vi "prepAO_tt.vi"() -> ()   [LabVIEW 2015]
uses:
  <vilib>/DAQmx/write.llb/DAQmx Write (Analog 1D Wfm NChan NSamp).vi
  <vilib>/DAQmx/create/channels.llb/DAQmx Create Channel (AO-Voltage-Basic).vi
  <vilib>/DAQmx/configure/timing.llb/DAQmx Timing (Sample Clock).vi
  <vilib>/DAQmx/miscellaneous.llb/DAQmx Fill In Error Info.vi
  <resource>/objmgr/daqmx.rc
panel:
  in  "error in 2":errorcluster caption="error in"
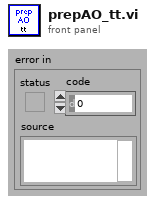
[diagram p1: front panel]
types:
  T1 = typedef "LVRectTypeDef.ctl" = cluster{"Left":i16, "Top":i16, "Right":i16, "Bottom":i16}
  T2 = cluster{"Xpixels":i32, "Vxminref":dbl, "Vxmaxref":dbl, "P":dbl, "Ypixels":i32, "Vyminref":dbl, "Vymaxref":dbl, "srate":sgl, "sAOxy":i32, "timeout":dbl, "type":string, "date":string, "time":string, "Colormap":u16, "Drawing Mode":u16, "Scanning Mode":u16, "square pixels":bool, "square matrix":bool, "Xpixels Img":i32, "Vx-min Img":dbl, "VX-max Img":dbl, "Ypixels Img":i32, "Vy-min Img":dbl, "Vy-max Img ":dbl, "Angle Img":dbl, "autoshutter":bool, "finite":bool, "cont":bool, "wavdet":bool, "measpoints":i32, "avpp":i32, "bufferAO":i32, "bufferAI":i32, "starttick":u32, "waveform":path, "Vx-ref":dbl, "Vy-ref":dbl, "refreshrate":dbl, "refreshbuffer":i32, "tt_cycles":i32, "motorref":refnum<k7>, "mirrorswitch":refnum<k7>, "sample mode":i32, "maxbufferAI":i32, "srateAODO":sgl, "bin":sgl, "Pel":sgl, "Angle draw":dbl, "srate Img":sgl, "ROIimg_plotbounds":T1, "auto OD":bool, "ODfilt":u16, "aAI":i32[], "aCI":i32[], "aAO":u32[], "aDO":u32[], "refwfsize":dbl, "Lifetime":bool, "Vz-Img":dbl, "Vz-ref":dbl, "Vz-reset":dbl, "AIoverride":bool}
  T3 = cluster{"StageS":i32, "StageL":i32, "currmeas data dir":path, "image OD":u16, "contour OD":u16, "point OD":u16, "AOlines":tag[], "AIlines":tag[], "CI lines":tag[], "DO lines":tag[], "AO names":string[], "CI names":string[], "AI names":string[], "DO names":string[], "CIextensions":string[], "AIextensions":string[], "Voltage to Ygalvo":i32, "Voltage to Xgalvo":i32, "Voltage to patch":i32, "640 shutter":i32, "2P shutter":i32, "LT timestamp":u32, "Vp":i32, "Ip":i32, "camera trigger":i32, "master data dir":path, "voltage to Zpos":i32, "Vto2P":i32, "640 AO":i32, "488 AO":i32, "532 AO":i32, "640TTL":u32, "488TTL":u32, "532TTL":u32}
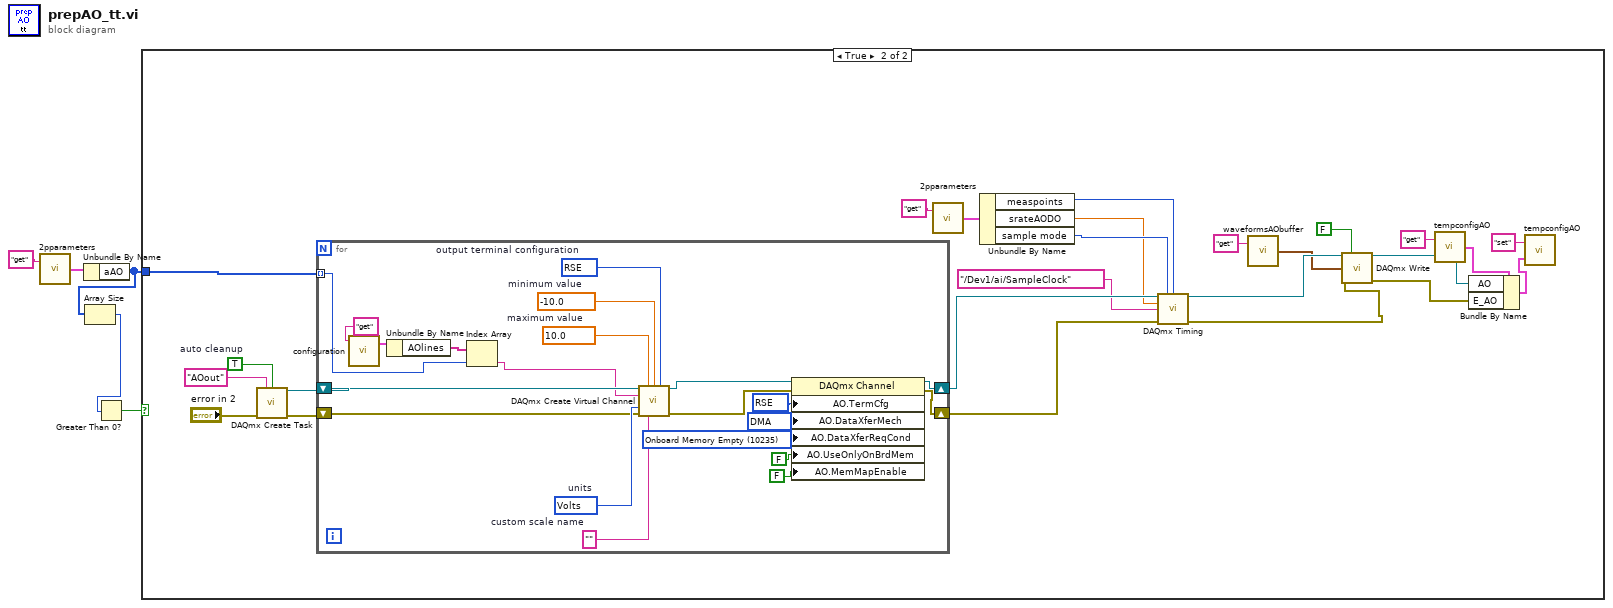
[diagram p0: block diagram]
diagram:
  n1 = call "2pparameters.vi"("command"="get") -> ("params out"=w4:T2)  [unwired: 1 in]
  n2 = Unbundle By Name(w4) -> ("aAO"=w1:u32[])
  n3 = Array Size(array=w1) -> (size(s)=w2:i32)
  n4 = Greater Than 0?(x=w2) -> (x > 0?=w3:bool)
  n5 = case shown="True" w3 {
    tunnel: w1 -> [_ w26]
    frame False {
    }
    frame True {
      w28 = TRUE  # auto cleanup
      n6 = call <vilib>:"DAQmx Create Task.vi"("new task name"="AOout", "auto cleanup"=w28, "error in"="error in 2") -> ("task out"=w29:refnum<k21>, "error out"=w30:errorcluster)  [unwired: 11 in]
      n7 = for {
        shift-right: [w33] -> w21
        shift-left: w29 -> [w47]
        shift-right: [w32] -> w20
        shift-left: w30 -> [w46]
        tunnel: w26 -> [w42] mode=indexing
        w37 = 10235 items=["Onboard Memory Empty"=10235, "Onboard Memory Half Full or Less"=10239, "Onboard Memory Less than Full"=10242] ("AO.DataXferReqCond 2")
        w38 = 10054 items=["DMA"=10054, "Interrupts"=10204, "Programmed I/O"=10264, "USB Bulk"=12590] ("AO.DataXferMech 2")
        w39 = 10083 items=["RSE"=10083, "Differential"=10106, "Pseudodifferential"=12529] ("AO.TermCfg")
        w51 = 10083 items=["Default"=-1, "RSE"=10083, "Differential"=10106, "Pseudodifferential"=12529]  # output terminal configuration
        w50 = 10348 items=["Volts"=10348, "From Custom Scale"=10065]  # units
        w40 = ""  # custom scale name
        w49 = -10.0  # minimum value
        w48 = 10.0  # maximum value
        n8 = call "configuration.vi"("command"="get") -> ("config out"=w43:T3)  [unwired: 2 in, 1 out]
        n9 = Unbundle By Name(w43) -> ("AOlines"=w45:tag[])
        n10 = Index Array(array=w45, index=w42) -> (element=w41:tag)
        n11 = call-poly <vilib>:"DAQmx Create Virtual Channel.vi"("task in"=w47, "maximum value"=w48, "minimum value"=w49, "output terminal configuration"=w51, "physical channels"=w41, "units"=w50, "error in"=w46, "custom scale name"=w40) -> ("task out"=w34:refnum<k21>, "error out"=w31:errorcluster)  [unwired: 6 in]
        n12 = property class="DAQmx Channel"(reference=w34, error in=w31, "AO.TermCfg"=w39, "AO.DataXferMech"=w38, "AO.DataXferReqCond"=w37, "AO.UseOnlyOnBrdMem"=FALSE, "AO.MemMapEnable"=FALSE) -> (reference out=w33:refnum<k21>, error out=w32:errorcluster)
      }
      n13 = call "2pparameters.vi"("command"="get") -> ("params out"=w23:T2)  [unwired: 1 in]
      n14 = Unbundle By Name(w23) -> ("measpoints"=w19:i32, "srateAODO"=w18:sgl, "sample mode"=w24:i32)
      n15 = call-poly <vilib>:"DAQmx Timing.vi"("task/channels in"=w21, "sample mode"=w24, "samples per channel"=w19, "rate"=w18, "source"=tag "/Dev1/ai/SampleClock", "error in"=w20) -> ("task out"=w10:refnum<k21>, "error out"=w9:errorcluster)  [unwired: 1 in, 7 out]
      n16 = call "waveformsAObuffer.vi"("command"="get") -> ("AO wf out"=w6:waveform(dbl)[])  [unwired: 1 in]
      n17 = call-poly <vilib>:"DAQmx Write.vi"("task/channels in"=w10, "auto start"=FALSE, "data"=w6, "error in"=w9) -> ("task out"=w11:refnum<k21>, "error out"=w12:errorcluster)  [unwired: 9 in, 1 out]
      n18 = call "tempconfigAO.vi"("command"="get") -> ("Temp Config out"=w14:cluster{"AO":refnum<k21>, "E_AO":errorcluster})  [unwired: 1 in]
      n19 = Bundle By Name(cluster=w14, "AO"=w11, "E_AO"=w12) -> (w13:cluster{"AO":refnum<k21>, "E_AO":errorcluster})
      n20 = call "tempconfigAO.vi"("Temp Config in"=w13, "command"="set") -> ()  [unwired: 1 out]
    }
  }
